vi "Get Category.vi"(8 "error in (no error)":errorcluster, 10 "Category Name":string, 11 "Database in":refnum<class "Account History.lvclass">) -> (0 "error out":errorcluster, 1 "Found?":bool, 2 "Category":refnum<class "Category.lvclass">, 3 "Database out":refnum<class "Account History.lvclass">)   [LabVIEW 2018, in "Account History.lvclass"]
uses:
  Account History.lvclass
  Category/Category.lvclass
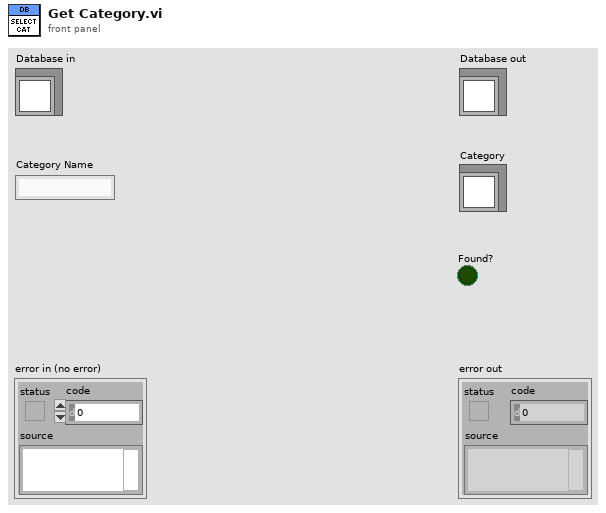
[diagram p1: front panel]
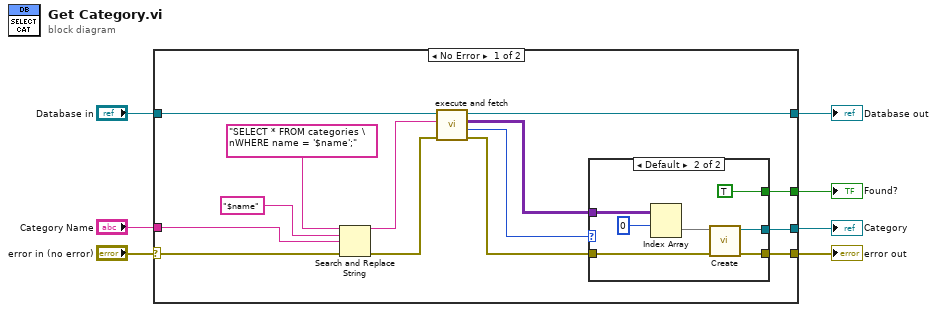
[diagram p0: block diagram]
diagram:
  n1 = case shown="No Error" "error in (no error)" {
    selector: "error in (no error)" -> [w13 w30]
    tunnel: "Database in" -> [w21 w31]
    tunnel: [w20 w31] -> w6
    tunnel: "Category Name" -> [w10 _]
    tunnel: [w18 w30] -> w4
    tunnel: [w16 _] -> w2
    tunnel: [w14 _] -> w1
    frame No Error {
      n2 = Search and Replace String(input string="SELECT * FROM categories \nWHERE name = '$name';", search string="$name", replace string=w10, error in=w13) -> (result string=w11:string, error out=w12:errorcluster)  [unwired: 4 in, 2 out]
      n3 = call "execute and fetch.vi"("error in (no error)"=w12, "SQL query"=w11, "Database in"=w21) -> ("error out"=w19:errorcluster, "Num records"=w15:i32, "recordset data"=w17:variant[][], "Database out"=w20:refnum<class "Account History.lvclass">)  [unwired: 5 in]
      n4 = case shown="Default" w15 {
        tunnel: w19 -> [w22 w29]
        tunnel: [w22 w28] -> w18
        tunnel: w17 -> [_ w27]
        tunnel: [_ w24] -> w16
        tunnel: [_ TRUE] -> w14
        frame 0 {
        }
        frame Default {
          n5 = Index Array(array=w27, index (row)=0) -> (element=w25:variant[])  [unwired: 1 in]
          n6 = call "Create.vi"("error in (no error)"=w29, "Record"=w25) -> ("error out"=w28:errorcluster, "Category out"=w24:refnum<class "Category.lvclass">)  [unwired: 8 in]
        }
      }
    }
    frame Error {
    }
  }
  "error out" <- w4
  "Database out" <- w6
  "Category" <- w2
  "Found?" <- w1
